vi "bylinear interpolation iiii- complex -- build matrix.vi"(11 "N":i32) -> (2 "Inverse Matrix":T1)   [LabVIEW 2020]
uses:
  <vilib>/Analysis/Matrix/Datatypes/RealMatrix.ctl
  <vilib>/Analysis/Matrix/Numeric/Conversions/Array To Matrix - RA2.vi
  <vilib>/Analysis/baseanly.llb/Real Inverse Matrix.vi
  <vilib>/Analysis/Matrix/NI_Matrix.lvlib
  <vilib>/Analysis/NI_AALBase.lvlib
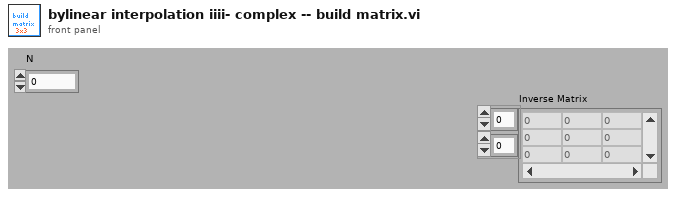
[diagram p1: front panel]
types:
  T1 = typedef "NI_Matrix.lvlib/RealMatrix.ctl" = dbl[][]
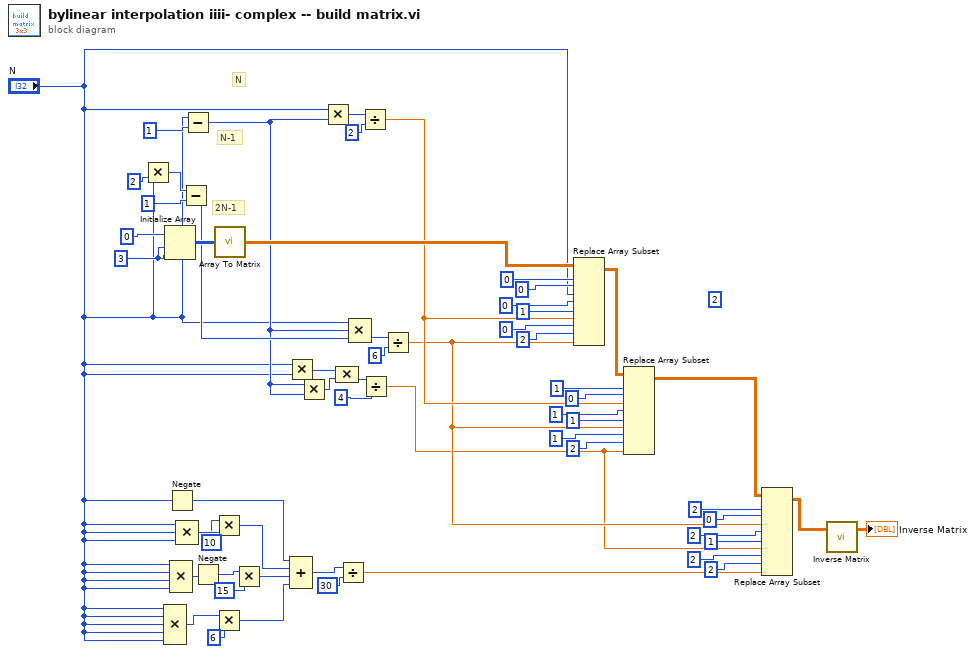
[diagram p0: block diagram]
diagram:
  (unwired) 2 ("n")
  w53 = 3 ("n")
  # "2N-1"
  # "N-1"
  # "N"
  n1 = Multiply(x="N", y=2 ("n")) -> (x*y=w55:i32)
  n2 = Compound Arithmetic op=MULTIPLY("N", "N", "N", "N", "N") -> (w6:i32)
  n3 = Initialize Array(0 ("n"), w53, w53) -> (w52:i32[][])
  n4 = Negate(x="N") -> (-x=w2:i32)
  n5 = Compound Arithmetic op=MULTIPLY("N", "N", "N", "N") -> (w17:i32)
  n6 = Compound Arithmetic op=MULTIPLY("N", "N", "N") -> (w14:i32)
  n7 = Subtract(x=w55, y=1 ("n")) -> (x-y=w44:i32)
  n8 = Subtract(x="N", y=1 ("n")) -> (x-y=w41:i32)
  n9 = Negate(x=w17) -> (-x=w10:i32)
  n10 = Multiply(x=10 ("n"), y=w14) -> (x*y=w11:i32)
  n11 = Multiply(x=w6, y=6 ("n")) -> (x*y=w5:i32)
  n12 = call-poly <vilib>:"Array To Matrix.vi"("Real 2D Array"=w52) -> ("Real Matrix"=w51:T1)
  n13 = Multiply(x=w10, y=15 ("n")) -> (x*y=w8:i32)
  n14 = Multiply(x="N", y="N") -> (x*y=w39:i32)
  n15 = Compound Arithmetic op=ADD(w2, w11, w8, w5) -> (w15:i32)
  n16 = Multiply(x=w41, y=w41) -> (x*y=w40:i32)
  n17 = Multiply(x="N", y=w41) -> (x*y=w48:i32)
  n18 = Compound Arithmetic op=MULTIPLY(w39, w40) -> (w42:i32)
  n19 = Divide(x=w15, y=30 ("n")) -> (x/y=w12:dbl)
  n20 = Compound Arithmetic op=MULTIPLY("N", w41, w44) -> (w45:i32)
  n21 = Divide(x=w48, y=2 ("n")) -> (x/y=w27:dbl)
  n22 = Divide(x=w42, y=4 ("n")) -> (x/y=w18:dbl)
  n23 = Divide(x=w45, y=6 ("n")) -> (x/y=w19:dbl)
  n24 = Replace Array Subset(array=w51, new element #1="N", index (row) #1=0 ("n"), index (col) #1=0 ("n"), new element #2=w27, index (row) #2=0 ("n"), index (col) #2=1 ("n"), new element #3=w19, index (row) #3=0 ("n"), index (col) #3=2 ("n")) -> (w28:T1)
  n25 = Replace Array Subset(array=w28, new element #1=w27, index (row) #1=1 ("n"), index (col) #1=0 ("n"), new element #2=w19, index (row) #2=1 ("n"), index (col) #2=1 ("n"), new element #3=w18, index (row) #3=1 ("n"), index (col) #3=2 ("n")) -> (w20:T1)
  n26 = Replace Array Subset(array=w20, new element #1=w19, index (row) #1=2 ("n"), index (col) #1=0 ("n"), new element #2=w18, index (row) #2=2 ("n"), index (col) #2=1 ("n"), new element #3=w12, index (row) #3=2 ("n"), index (col) #3=2 ("n")) -> (w4:T1)
  n27 = call-poly <vilib>:"Inverse Matrix.vi"("Input Matrix"=w4) -> ("Inverse Matrix"=→"Inverse Matrix":T1)  [unwired: 1 in, 1 out]
